vi "M14_Hardware_Spindexer_Globals.vi"() -> ()   [LabVIEW 2019]
panel:
  in  "Spindexer":string="Spindexer"
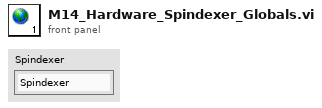
[diagram p1: front panel]
diagram:
